vi "ArmFF_MinAchieveAccel.vi"(8 "Velocity":dbl, 9 "Angle":dbl, 10 "MaxVoltage":dbl, 11 "in ARM_FF":T1 {"kCos" format="%13.5p"; "Ka" format="%13.5p"; "Kv" format="%13.5p"; "Ks" format="%13.5p"}) -> (3 "MinAccel":dbl)   [LabVIEW 2019, in "Trajectory_Library.lvlib"]
doc: "Calculates the minimum achievable acceleration given a maximum voltage supply, a position, and a velocity. Useful for ensuring that velocity and acceleration constraints for a trapezoidal profile are simultaneously achievable - enter the velocity constraint, and this will give you a simultaneously-achievable acceleration constraint.\n \nInputs: \n - ArmFF -- The ArmFF data cluster\n - maxVoltage -- The maximum voltage that can be supplied to the arm.\n - angle -- The angle of the arm.\n - velocity -- The velocity of the arm.\n\nOutputs:\n - MinAccel -- The minimum possible acceleration at the given velocity."
uses:
  Trajectory_Library.lvlib
  TypeDef/ARM_FF.ctl
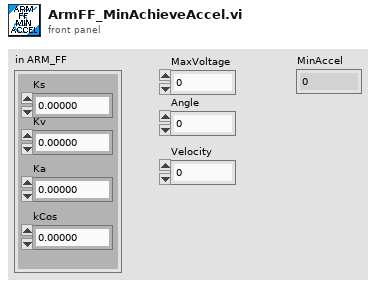
[diagram p1: front panel]
types:
  T1 = typedef "Trajectory_Library.lvlib/ARM_FF.ctl" = cluster{"Ks":dbl, "Kv":dbl, "Ka":dbl, "kCos":dbl}
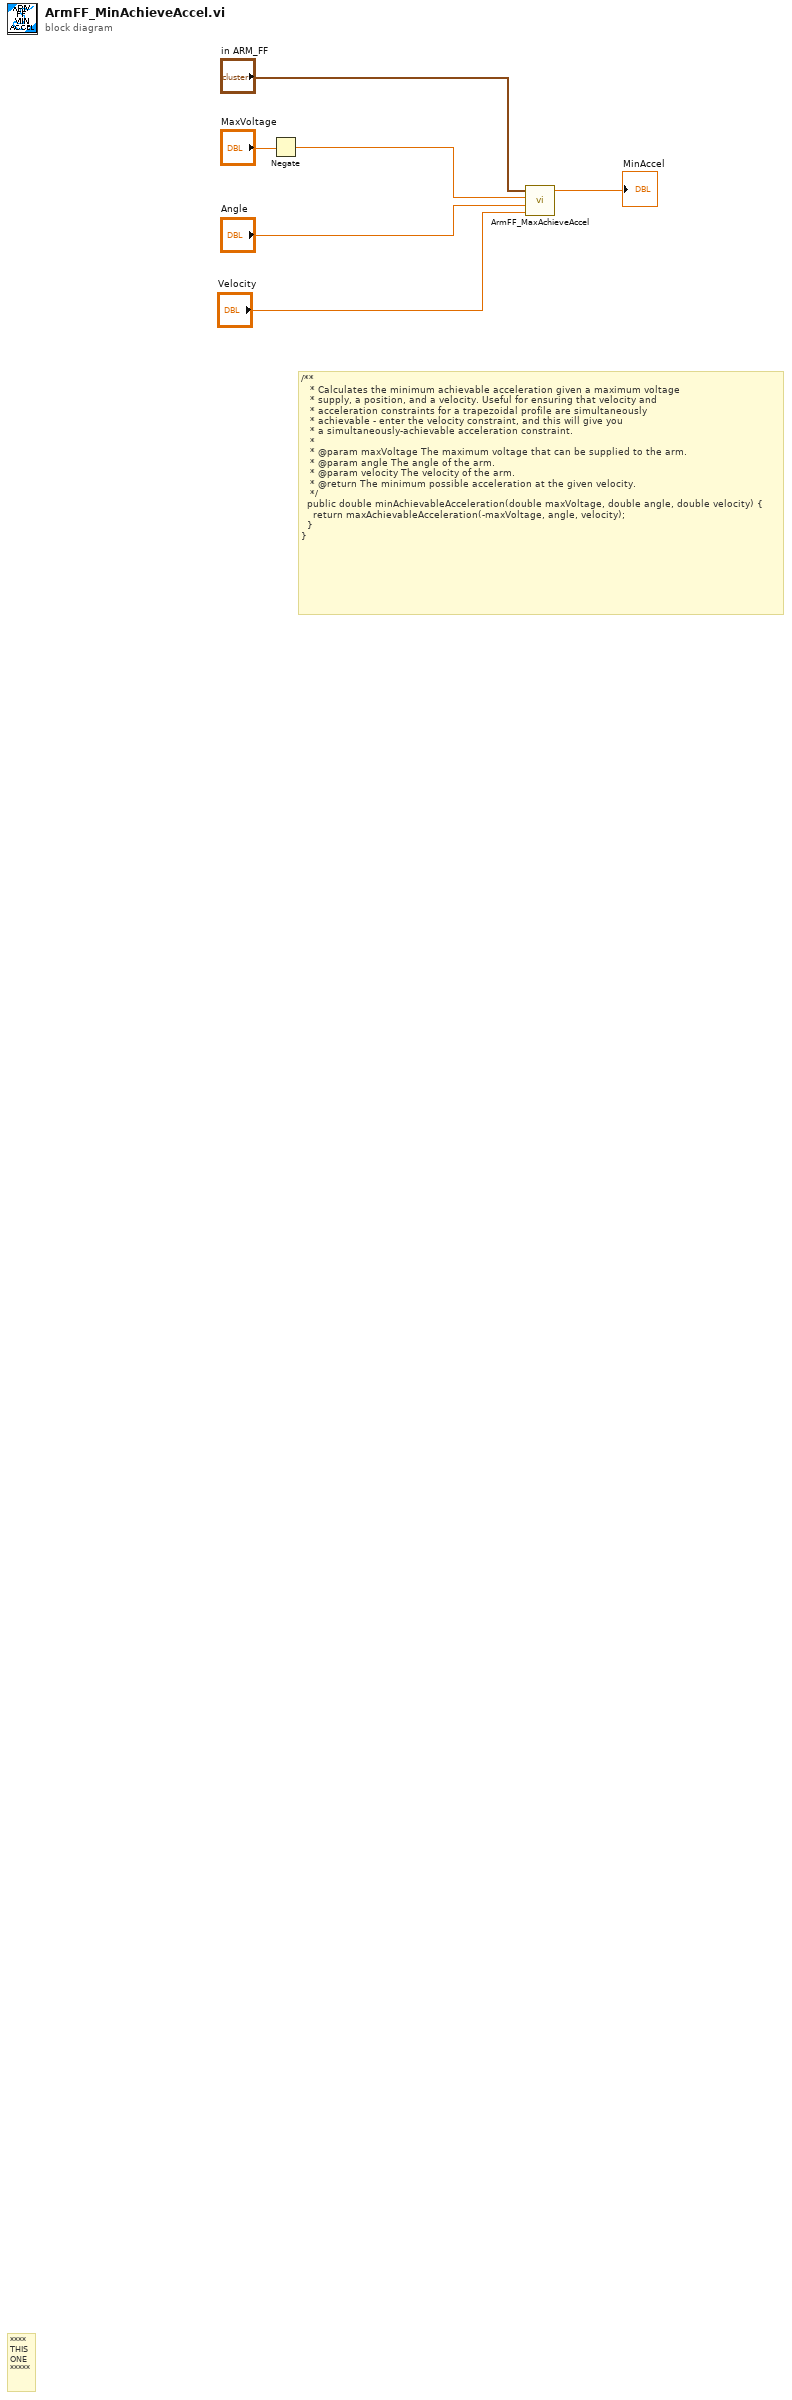
[diagram p0: block diagram]
diagram:
  # "/**\n   * Calculates the minimum achievable acceleration given a maximum voltage\n   * supply, a position, and a velocity. Useful for ensuring that velocity and\n   * acceleration constraints for a trapezoidal profile are simultaneously\n   * achievable - enter the velocity constraint, and this will give you\n   * a simultaneously-achievable acceleration constraint.\n   *\n   * @param maxVoltage The maximum voltage that can be supplied to the arm.\n   * @param angle The angle of the arm.\n   * @param velocity The velocity of the arm.\n   * @return The minimum possible acceleration at the given velocity.\n   */\n  public double minAchievableAcceleration(double maxVoltage, double angle, double velocity) {\n    return maxAchievableAcceleration(-maxVoltage, angle, velocity);\n  }\n}"
  # "****\nTHIS\nONE\n*****"
  n1 = Negate(x="MaxVoltage") -> (-x=w4:dbl)
  n2 = call "ArmFF_MaxAchieveAccel.vi"("Velocity"="Velocity", "Angle"="Angle", "MaxVoltage"=w4, "in ARM_FF"="in ARM_FF") -> ("MaxAccel"=→"MinAccel":dbl)  [unwired: 7 in]
